vi "PV ActiveLine - Convert Data.vi"(11 "String in":string) -> (0 "DBL out":dbl[](array[numeric]), 1 "Integer Out":i32[](array[numeric]), 2 "Read Status":u16(ring) items=["Read Failed", "Read Ok"], 3 "String out":string[](array[string]))   [LabVIEW 2013, in "PV ActiveLine.lvlib"]
uses:
  PV ActiveLine.lvlib
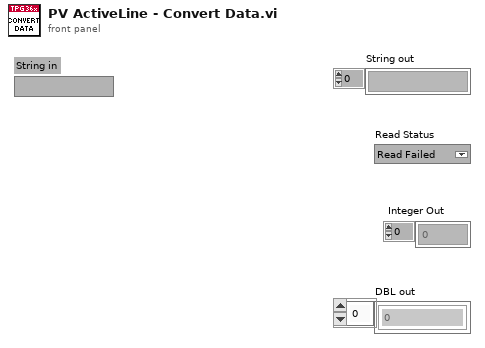
[diagram p1: front panel]
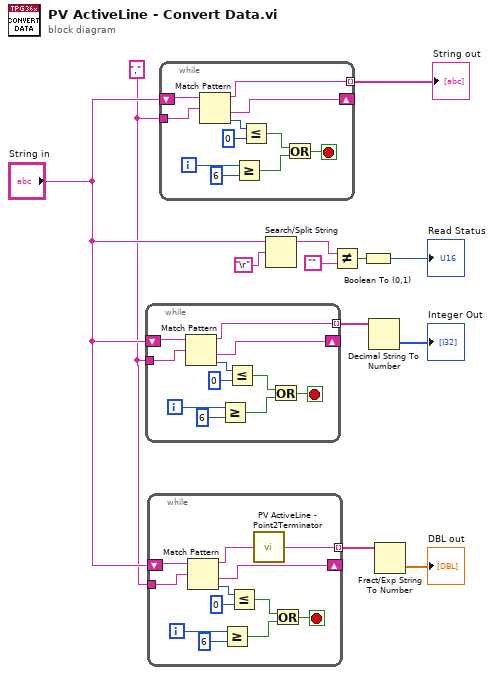
[diagram p0: block diagram]
diagram:
  w2 = "," ("regular expression")
  n1 = while {
    shift-right: [w15] -> _
    shift-left: "String in" -> [w17]
    tunnel: [w16] -> w10 mode=indexing
    tunnel: w2 -> [w13]
    i -> [w18]
    stop <- w19 stop-if-true
    n2 = Match Pattern(string=w17, regular expression=w13) -> (before substring=w16:string, after substring=w15:string, offset past match=w14:i32)  [unwired: 1 in, 1 out]
    n3 = Greater Or Equal?(x=w18, y=6 ("x")) -> (x >= y?=w20:bool)
    n4 = Less Or Equal?(x=w14, y=0) -> (x <= y?=w21:bool)
    n5 = Or(x=w21, y=w20) -> (x .or. y?=w19:bool)
  }
  n6 = while {
    shift-right: [w28] -> _
    shift-left: "String in" -> [w29]
    tunnel: [w24] -> w9 mode=indexing
    tunnel: w2 -> [w26]
    i -> [w30]
    stop <- w31 stop-if-true
    n7 = Match Pattern(string=w29, regular expression=w26) -> (before substring=w25:string, after substring=w28:string, offset past match=w27:i32)  [unwired: 1 in, 1 out]
    n8 = Greater Or Equal?(x=w30, y=6 ("x")) -> (x >= y?=w32:bool)
    n9 = Less Or Equal?(x=w27, y=0) -> (x <= y?=w33:bool)
    n10 = call "PV ActiveLine - Point2Terminator.vi"("Eingangstring"=w25) -> ("Ausgangstring"=w24:string)
    n11 = Or(x=w33, y=w32) -> (x .or. y?=w31:bool)
  }
  n12 = while {
    shift-right: [w38] -> _
    shift-left: "String in" -> [w40]
    tunnel: [w39] -> w1 mode=indexing
    tunnel: w2 -> [w36]
    i -> [w41]
    stop <- w42 stop-if-true
    n13 = Match Pattern(string=w40, regular expression=w36) -> (before substring=w39:string, after substring=w38:string, offset past match=w37:i32)  [unwired: 1 in, 1 out]
    n14 = Greater Or Equal?(x=w41, y=6 ("x")) -> (x >= y?=w43:bool)
    n15 = Less Or Equal?(x=w37, y=0) -> (x <= y?=w44:bool)
    n16 = Or(x=w44, y=w43) -> (x .or. y?=w42:bool)
  }
  "String out" <- w1
  n17 = Search/Split String(string="String in", search string/char (-)="\r") -> (substring before match=w4:string)  [unwired: 1 in, 2 out]
  n18 = Not Equal?(x=w4, y="") -> (x != y?=w6:bool)
  n19 = Boolean To (0,1)(Boolean=w6) -> (0, 1=→"Read Status":i16)
  n20 = Decimal String To Number(string=w10) -> (number=→"Integer Out":i32[])  [unwired: 2 in, 1 out]
  n21 = Fract/Exp String To Number(string=w9) -> (number=→"DBL out":dbl[])  [unwired: 3 in, 1 out]
